vi "User Settings.vi"() -> ()   [LabVIEW 2025]
doc: "Access Level Admin only.\nFeature supported:\n1.Add User\n2.Change Password\n3.Remove User"
uses:
  <vilib>/addons/database/Connection.llb/Conn ObjectReference.ctl
  <vilib>/Utility/miscctls.llb/LVRectTypeDef.ctl
  <vilib>/Utility/error.llb/Trim Whitespace One-Sided.vi
  <vilib>/addons/database/NI_Database_API.lvlib
panel:
  in  "error in":errorcluster
  in  "User Configuration":string(tree)
  in  "Exit":bool
  in  "User Mangement":enum32{"Add", "Edit", "Delete"}(radio)
  in  "User_Tab":enum32{"Add", "Edit", "Delete"}(tab)
  in  "Add User":bool
  in  "Work Group":string(combo)="Operator"
  in  "Confirm Password":string
  in  "New Password":string
  in  "New User":string
  out "UserName Edit":string caption="UserName"
  in  "ChangeCONFIRMPassword":string caption="Confirm Password *"
  in  "ChangeNEWPassword":string caption="New Password *"
  in  "ChangeOldPassword":string caption="Current Password *"
  in  "Update User":bool
  in  "Remove User":bool
  out "UserName Delete":string caption="UserName"
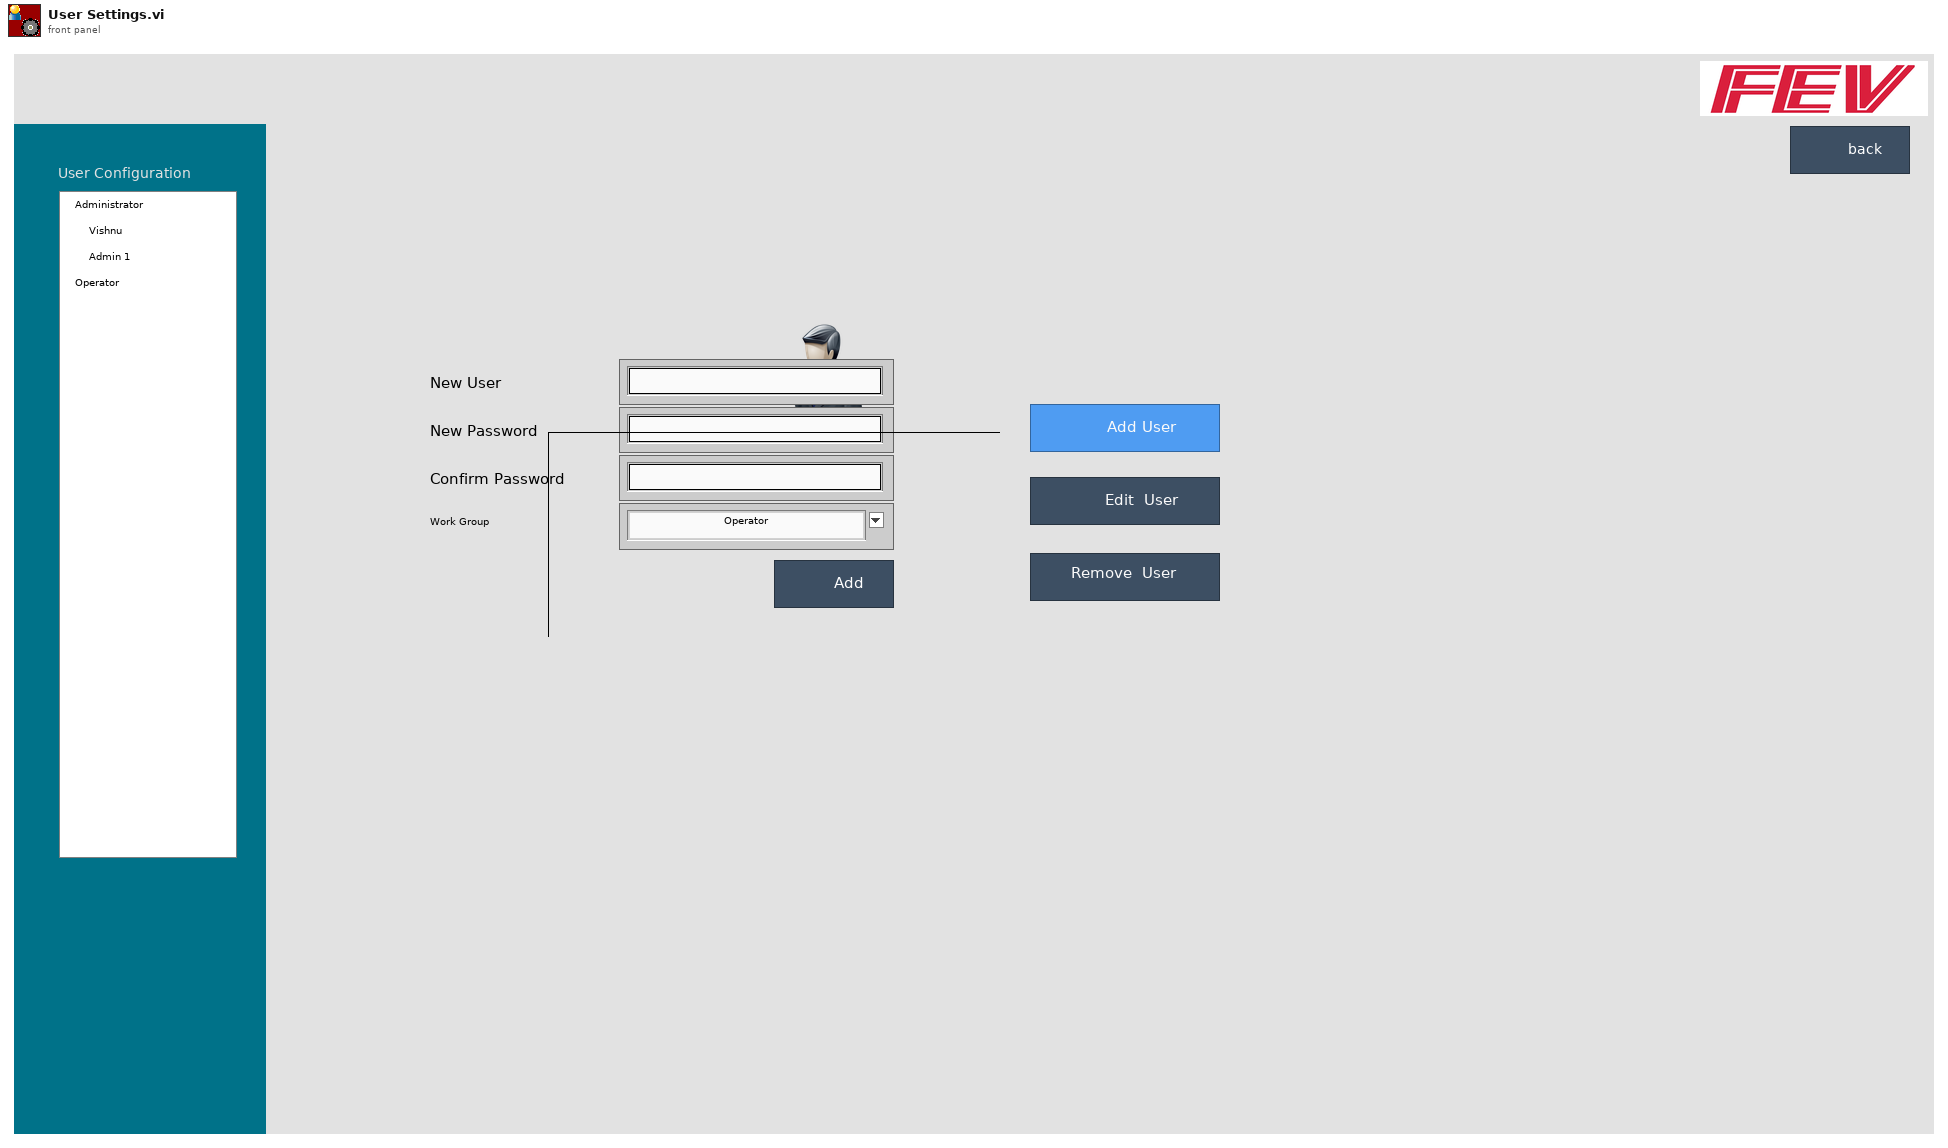
[diagram p1: front panel]
types:
  T1 = typedef "LVRectTypeDef.ctl" = cluster{"Left":i16, "Top":i16, "Right":i16, "Bottom":i16}
  T2 = typedef "NI_Database_API.lvlib/Conn ObjectReference.ctl" = refnum<k1>
  T3 = cluster{"UserDetails":string[][], "AcitveDBCon":T2}
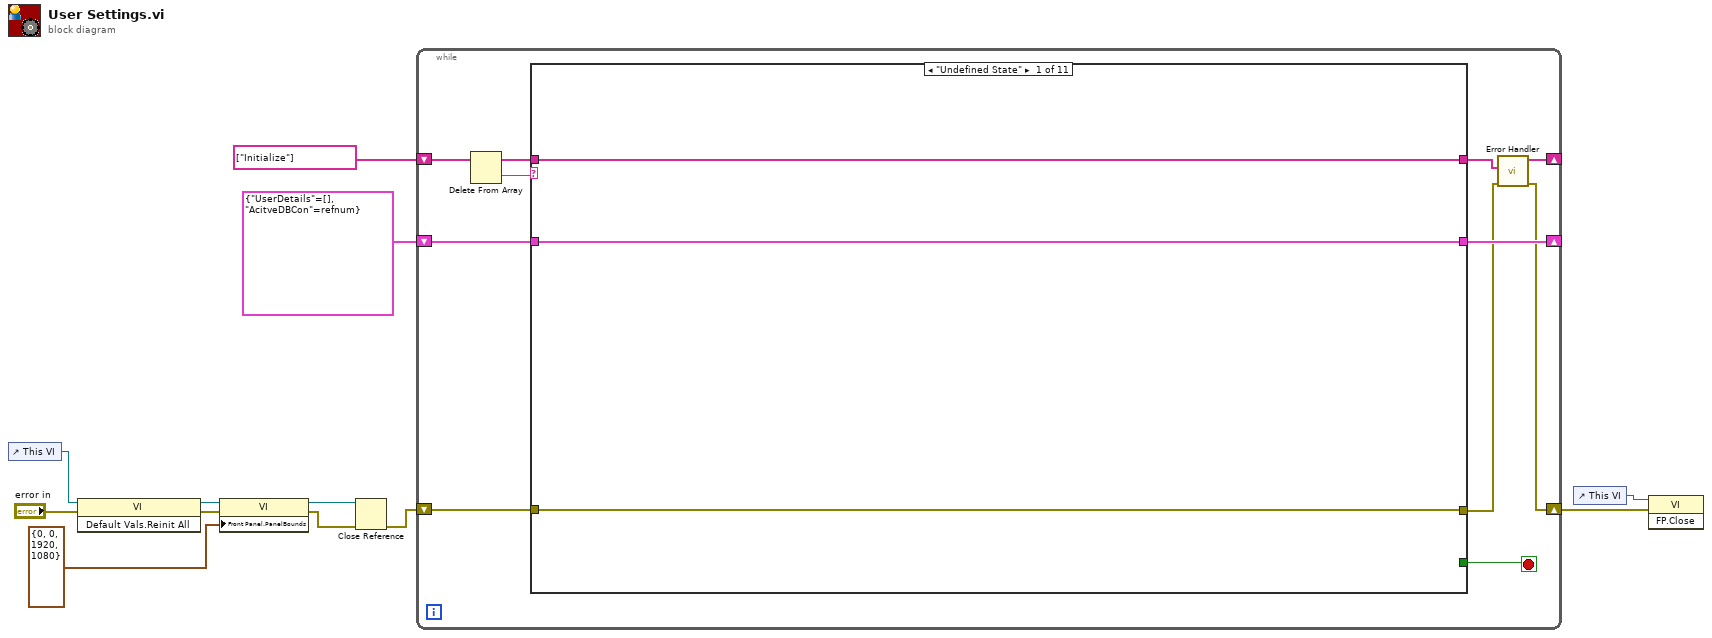
[diagram p0: block diagram]
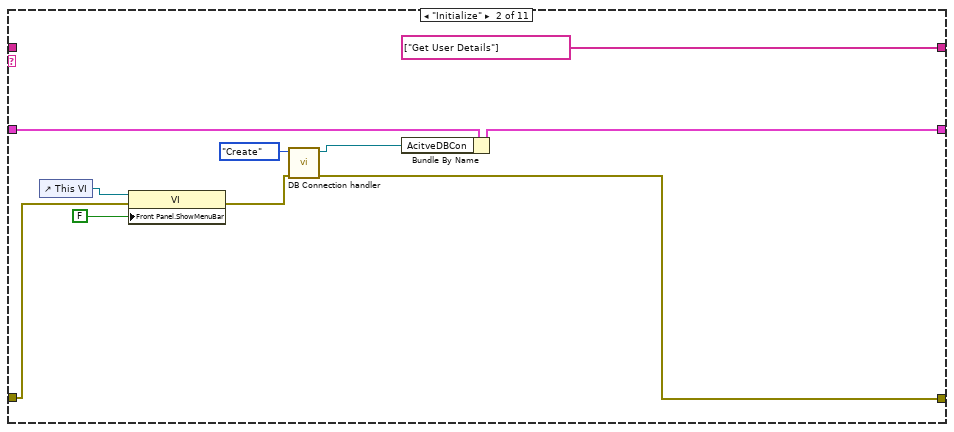
[diagram p2: hidden frame]
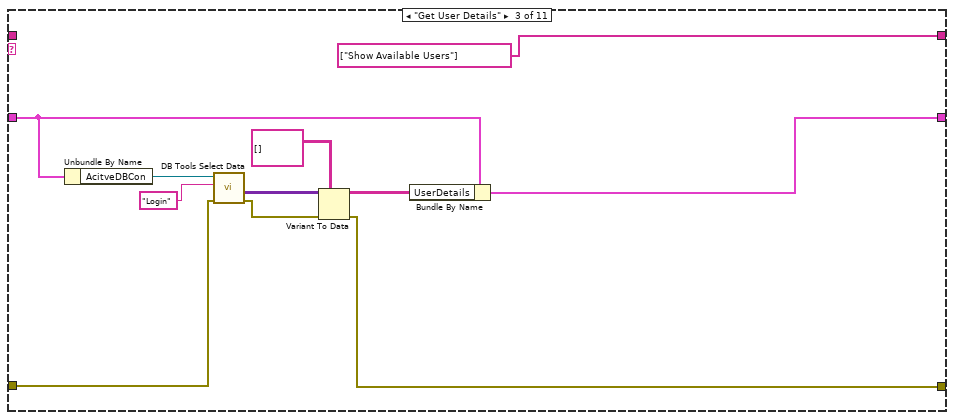
[diagram p3: hidden frame]
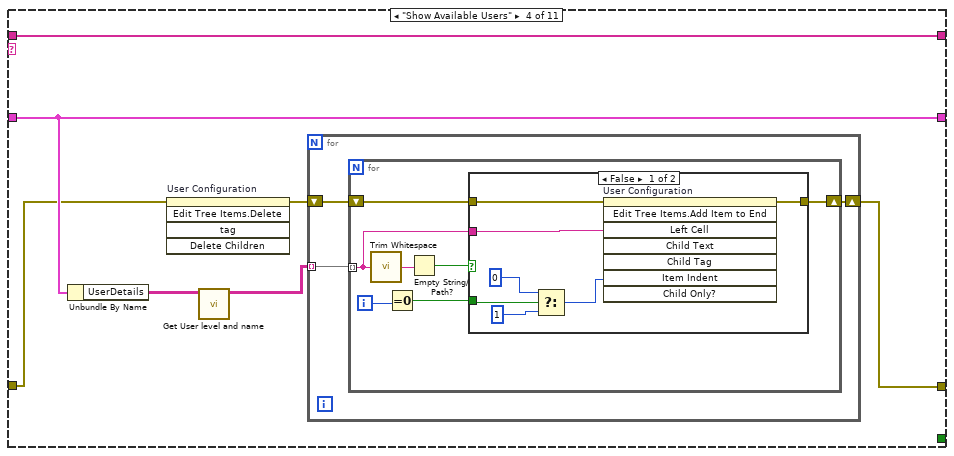
[diagram p4: hidden frame]
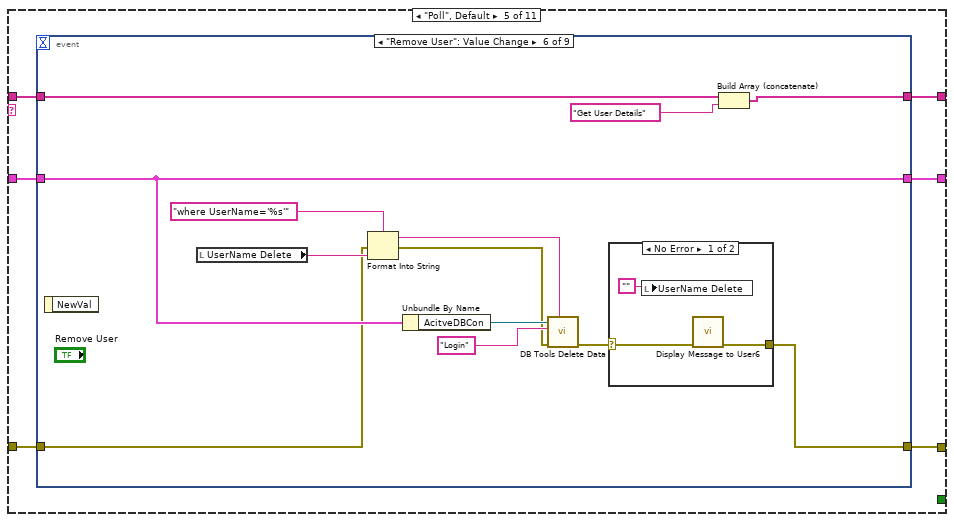
[diagram p6: hidden frame]
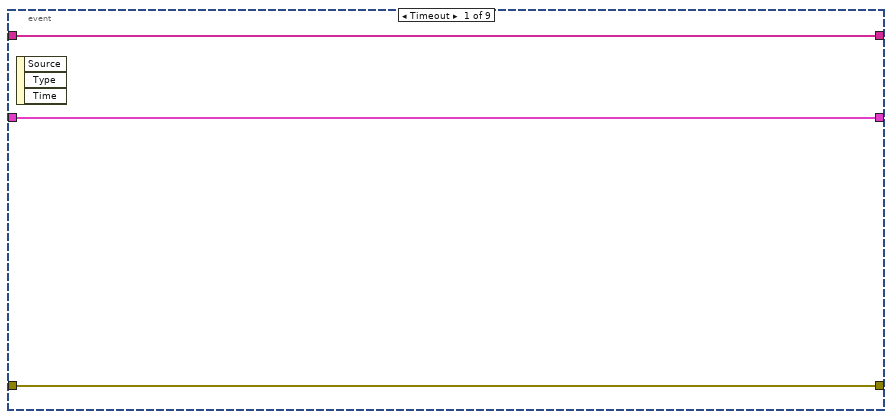
[diagram p7: hidden frame]
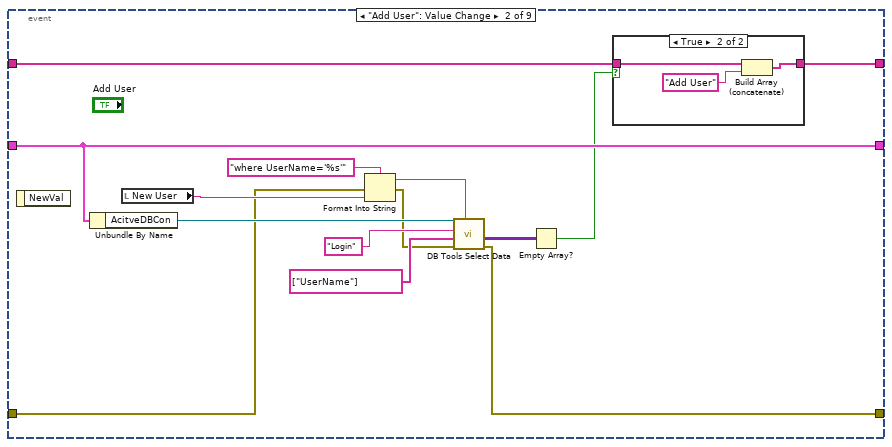
[diagram p8: hidden frame]
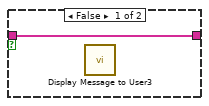
[diagram p9: hidden frame]
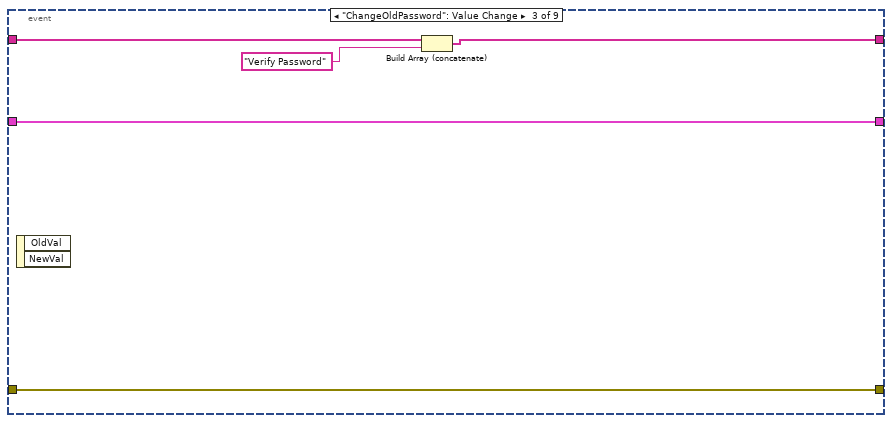
[diagram p10: hidden frame]
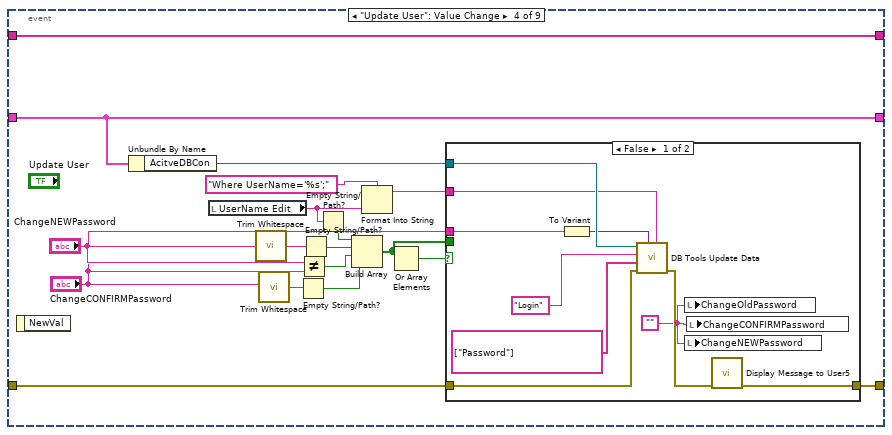
[diagram p11: hidden frame]
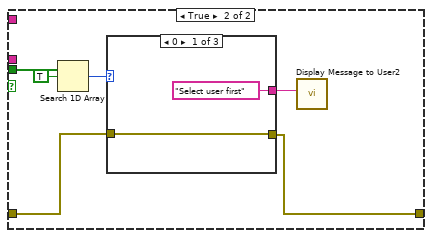
[diagram p12: hidden frame]
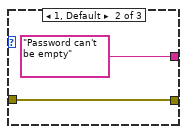
[diagram p13: hidden frame]
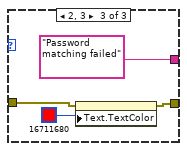
[diagram p14: hidden frame]
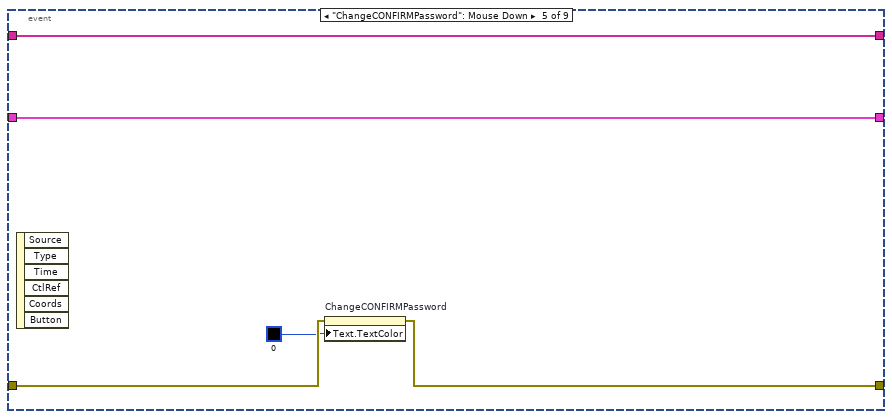
[diagram p15: hidden frame]
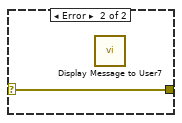
[diagram p16: hidden frame]
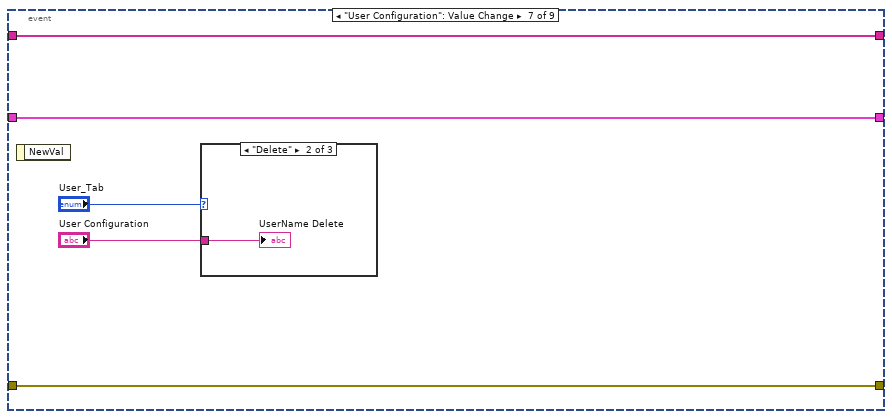
[diagram p17: hidden frame]
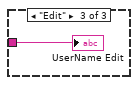
[diagram p19: hidden frame]
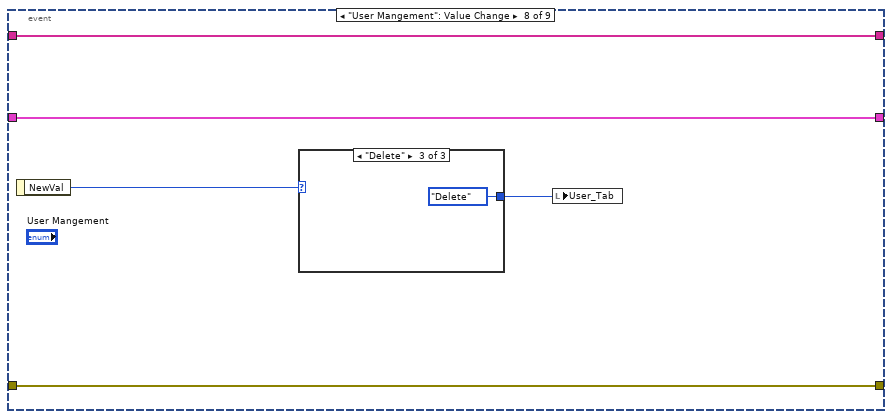
[diagram p20: hidden frame]
diagram:
  n1 = control-ref of="This VI"() -> (w6:refnum<vi>)
  n2 = invoke class="VI" method="Default Vals.Reinit All"(reference=w6, error in="error in") -> (reference out=w5:refnum<vi>, error out=w2:errorcluster)  [unwired: 1 in, 1 out]
  n3 = property class="VI"(reference=w5, error in=w2, "Front Panel.PanelBounds"=T1 {"Left"=0, "Top"=0, "Right"=1920, "Bottom"=1080} ("Front Panel Window:Window Bounds")) -> (reference out=w4:refnum<vi>, error out=w1:errorcluster)
  n4 = Close Reference(reference=w4, error in (no error)=w1) -> (error out=w11:errorcluster)
  n5 = while {
    shift-right: [w17] -> _
    shift-left: string[] ["Initialize"] -> [w22]
    shift-right: [w20] -> _
    shift-left: T3 {"UserDetails"=[], "AcitveDBCon"=refnum} -> [w19]
    shift-right: [w15] -> w7
    shift-left: w11 -> [w18]
    stop <- w14 stop-if-true
    n6 = Delete From Array(array=w22) -> (deleted portion=w23:string, array with subset deleted=w21:string[])  [unwired: 2 in]
    n7 = case shown="\"Undefined State\"" w23 {
      tunnel: [w26 string[] ["Get User Details"] string[] ["Show Available Users"] w54 w76 w192 w205 w223 w225 w240 w244] -> w13
      tunnel: w21 -> [w26 _ _ w54 w75 w200 w205 w223 w233 w240 w244]
      tunnel: [w25 w33 w46 w52 w78 w199 w217 w222 w232 w239 w243] -> w20
      tunnel: w19 -> [w25 w35 w45 w52 w77 w199 w217 w222 w232 w239 w243]
      tunnel: w18 -> [w24 w28 w38 w50 w73 w197 w213 w221 w227 w236 w241]
      tunnel: [w24 w31 w37 w53 w74 w189 w207 w221 w226 w234 w241] -> w16
      tunnel: [_ _ _ _ _ _ _ _ _ TRUE TRUE] -> w14
      frame "Undefined State" {
      }
      frame "Initialize" {
        n8 = control-ref of="This VI"() -> (w30:refnum<vi>)
        n9 = property class="VI"(reference=w30, error in=w28, "Front Panel.ShowMenuBar"=FALSE ("Front Panel Window:Show Menu Bar")) -> (error out=w27:errorcluster)  [unwired: 1 out]
        n10 = call "DB Connection handler.vi"("error in (no error)"=w27, "DB Action"=enum16{"Create", "Close", "Get"}."Create") -> ("error out"=w31:errorcluster, "connection reference"=w32:T2)  [unwired: 8 in]
        n11 = Bundle By Name(cluster=w35, "AcitveDBCon"=w32) -> (w33:T3)
      }
      frame "Get User Details" {
        n12 = Unbundle By Name(w45) -> ("AcitveDBCon"=w44:T2)
        n13 = call <vilib>:"DB Tools Select Data.vi"("error in (no error)"=w38, "table"="Login", "connection reference"=w44) -> ("error out"=w39:errorcluster, "data"=w41:variant[][])  [unwired: 3 in, 1 out]
        n14 = Variant To Data(error in=w39, type=string[][] [], Variant=w41) -> (data=w40:string[][], error out=w37:errorcluster)
        n15 = Bundle By Name(cluster=w45, "UserDetails"=w40) -> (w46:T3)
      }
      frame "Show Available Users" {
        n16 = Unbundle By Name(w52) -> ("UserDetails"=w49:string[][])
        n17 = invoke on="User Configuration" class="Tree (strict)" method="Edit Tree Items.Delete"(error in=w50) -> (error out=w51:errorcluster)  [unwired: 4 in, 4 out]
        n18 = call "Get User level and name.vi"("UserDetails"=w49) -> ("UserL&N"=w48:string[][])  [unwired: 10 in]
        n19 = for {
          tunnel: w48 -> [w55] mode=indexing
          shift-right: [w57] -> w53
          shift-left: w51 -> [w56]
          n20 = for {
            shift-right: [w64] -> w57
            shift-left: w56 -> [w63]
            tunnel: w55 -> [w60] mode=indexing
            i -> [w62]
            n21 = call <vilib>:"Trim Whitespace.vi"("string"=w60) -> ("trimmed string"=w59:string)  [unwired: 1 in]
            n22 = Equal To 0?(x=w62) -> (x = 0?=w61:bool)
            n23 = Empty String/Path?(string/path=w59) -> (empty?=w58:bool)
            n24 = case shown="False" w58 {
              tunnel: [w71 w72] -> w64
              tunnel: w63 -> [w70 w72]
              tunnel: w61 -> [w69 _]
              tunnel: w60 -> [w65 _]
              frame False {
                n25 = Select(t=0, s=w69, f=1) -> (s? t:f=w66:i32)
                n26 = invoke on="User Configuration" class="Tree (strict)" method="Edit Tree Items.Add Item to End"(error in=w70, "Left Cell"=w65, "Item Indent"=w66) -> (error out=w71:errorcluster)  [unwired: 5 in, 7 out]
              }
              frame True {
              }
            }
          }
        }
      }
      frame "Poll", Default {
        n27 = event shown="[5] \"Remove User\": Value Change" {
          selector: _ -> [_ _ _ _ _ _ _ _ _]
          dyn-events: _ -> [_ _ _ _ _ _ _ _ _]
          timeout: _ -> [_ _ _ _ _ _ _ _ _]
          tunnel: [w81 w93 w104 w118 w150 w163 w172 w178 w187] -> w78
          tunnel: w77 -> [w81 w93 w104 w118 w150 w163 w172 w178 w187]
          tunnel: [w80 w95 w103 w122 w151 w155 w173 w179 w185] -> w76
          tunnel: w75 -> [w80 w94 w100 w122 w151 w164 w173 w179 w188]
          tunnel: [w79 w84 w101 w115 w148 w152 w171 w180 w186] -> w74
          tunnel: w73 -> [w79 w86 w101 w116 w149 w157 w171 w180 w186]
          event Timeout {
            n28 = event-data() -> ()  [unwired: 1 in, 3 out]
          }
          event "Add User": Value Change {
            n29 = event-data() -> ()  [unwired: 1 in, 1 out]
            n30 = Unbundle By Name(w93) -> ("AcitveDBCon"=w92:T2)
            n31 = local read "New User"() -> (w88:string)
            n32 = Format Into String(format string="where UserName='%s'", error in=w86, w88) -> (resulting string=w87:string, error out=w85:errorcluster)  [unwired: 1 in]
            n33 = call <vilib>:"DB Tools Select Data.vi"("condition"=w87, "error in (no error)"=w85, "columns"=string[] ["UserName"], "table"="Login", "connection reference"=w92) -> ("error out"=w84:errorcluster, "data"=w83:variant[][])  [unwired: 1 in, 1 out]
            n34 = Empty Array?(array=w83) -> (empty?=w82:bool)
            n35 = case shown="True" w82 {
              tunnel: [w96 w99] -> w95
              tunnel: w94 -> [w96 w97]
              frame False {
                n36 = call "Display Message to User3"() -> ()  [unwired: 10 in, 2 out]
              }
              frame True {
                n37 = Build Array (concatenate)(w97, "Add User") -> (w99:string[])
              }
            }
          }
          event "ChangeOldPassword": Value Change {
            n38 = event-data() -> ()  [unwired: 1 in, 2 out]
            n39 = Build Array (concatenate)(w100, "Verify Password") -> (w103:string[])
          }
          event "Update User": Value Change {
            n40 = event-data() -> ()  [unwired: 1 in, 1 out]
            n41 = Unbundle By Name(w118) -> ("AcitveDBCon"=w117:T2)
            n42 = local read "UserName Edit"() -> (w105:string)
            n43 = call <vilib>:"Trim Whitespace.vi"("string"="ChangeNEWPassword") -> ("trimmed string"=w121:string)  [unwired: 1 in]
            n44 = call <vilib>:"Trim Whitespace.vi"("string"="ChangeCONFIRMPassword") -> ("trimmed string"=w120:string)  [unwired: 1 in]
            n45 = Empty String/Path?(string/path=w120) -> (empty?=w109:bool)
            n46 = Not Equal?(x="ChangeNEWPassword", y="ChangeCONFIRMPassword") -> (x != y?=w110:bool)
            n47 = Empty String/Path?(string/path=w121) -> (empty?=w111:bool)
            n48 = Empty String/Path?(string/path=w105) -> (empty?=w106:bool)
            n49 = Build Array(w106, w111, w110, w109) -> (w107:bool[])
            n50 = Format Into String(format string="Where UserName='%s';", w105) -> (resulting string=w113:string)  [unwired: 2 in, 1 out]
            n51 = Or Array Elements(Boolean array=w107) -> (logical OR=w108:bool)
            n52 = case shown="False" w108 {
              tunnel: w117 -> [w132 _]
              tunnel: w116 -> [w129 w134]
              tunnel: [w124 w133] -> w115
              tunnel: "ChangeCONFIRMPassword" -> [w128 _]
              tunnel: w113 -> [w127 _]
              tunnel: w107 -> [_ w138]
              frame False {
                w123 = ""
                n53 = To Variant(anything=w128) -> (Variant=w126:variant)
                n54 = call <vilib>:"DB Tools Update Data.vi"("condition"=w127, "data"=w126, "error in (no error)"=w129, "columns"=string[] ["Password"], "table"="Login", "connection reference"=w132) -> ("error out"=w125:errorcluster)  [unwired: 4 in, 1 out]
                n55 = local write "ChangeOldPassword"(w123) -> ()
                n56 = local write "ChangeNEWPassword"(w123) -> ()
                n57 = local write "ChangeCONFIRMPassword"(w123) -> ()
                n58 = call "Display Message to User5"("error in (no error)"=w125) -> ("error out"=w124:errorcluster)  [unwired: 9 in, 1 out]
              }
              frame True {
                n59 = Search 1D Array(1D array=w138, element=TRUE) -> (index of element=w136:i32)  [unwired: 1 in]
                n60 = case shown="0" w136 {
                  tunnel: ["Select user first" "Password can't be empty" "Password matching failed"] -> w135
                  tunnel: w134 -> [w140 w141 w144]
                  tunnel: [w140 w141 w143] -> w133
                  frame 0 {
                  }
                  frame 1, Default {
                  }
                  frame 2, 3 {
                    n61 = property on="ChangeCONFIRMPassword" class="Str"(error in=w144, "Text.TextColor"=u32 16711680) -> (error out=w143:errorcluster)  [unwired: 1 in, 1 out]
                  }
                }
                n62 = call "Display Message to User2"("Message"=w135) -> ()  [unwired: 9 in, 2 out]
              }
            }
          }
          event "ChangeCONFIRMPassword": Mouse Down {
            n63 = event-data() -> ()  [unwired: 1 in, 6 out]
            n64 = property on="ChangeCONFIRMPassword" class="Str"(error in=w149, "Text.TextColor"=u32 0) -> (error out=w148:errorcluster)  [unwired: 1 in, 1 out]
          }
          event "Remove User": Value Change {
            n65 = event-data() -> ()  [unwired: 1 in, 1 out]
            n66 = local read "UserName Delete"() -> (w159:string)
            n67 = Format Into String(format string="where UserName='%s'" ("condition"), error in=w157, w159) -> (resulting string=w158:string, error out=w156:errorcluster)  [unwired: 1 in]
            n68 = Unbundle By Name(w163) -> ("AcitveDBCon"=w162:T2)
            n69 = call <vilib>:"DB Tools Delete Data.vi"("condition"=w158, "error in (no error)"=w156, "table"="Login", "connection reference"=w162) -> ("error out"=w153:errorcluster)  [unwired: 6 in, 1 out]
            n70 = case shown="No Error" w153 {
              selector: w153 -> [w167 w168]
              tunnel: [w166 w168] -> w152
              frame No Error {
                n71 = local write "UserName Delete"("") -> ()
                n72 = call "Display Message to User6"("error in (no error)"=w167) -> ("error out"=w166:errorcluster)  [unwired: 9 in, 1 out]
              }
              frame Error {
                n73 = call "Display Message to User7"() -> ()  [unwired: 10 in, 2 out]
              }
            }
            n74 = Build Array (concatenate)(w164, "Get User Details") -> (w155:string[])
          }
          event "User Configuration": Value Change {
            n75 = event-data() -> ()  [unwired: 1 in, 1 out]
            n76 = case shown="\"Delete\"" "User_Tab" {
              tunnel: "User Configuration" -> [_ w174 w175]
              frame "Add", Default {
              }
              frame "Delete" {
                "UserName Delete" <- w174
              }
              frame "Edit" {
                "UserName Edit" <- w175
              }
            }
          }
          event "User Mangement": Value Change {
            n77 = event-data() -> ("NewVal"=w177:enum32{"Add", "Edit", "Delete"})  [unwired: 1 in]
            n78 = case shown="\"Delete\"" w177 {
              tunnel: [enum32{"Add", "Edit", "Delete"}."Add" ("User_Tab") enum32{"Add", "Edit", "Delete"}."Edit" ("User_Tab") enum32{"Add", "Edit", "Delete"}."Delete" ("User_Tab")] -> w176
              frame "Add", Default {
              }
              frame "Edit" {
              }
              frame "Delete" {
              }
            }
            n79 = local write "User_Tab"(w176) -> ()
          }
          event "Exit": Value Change {
            n80 = event-data() -> ()  [unwired: 1 in, 6 out]
            n81 = Build Array (concatenate)(w188, "Exit") -> (w185:string[])
          }
        }
      }
      frame "Add User" {
        n82 = Unbundle By Name(w199) -> ("AcitveDBCon"=w198:T2)
        n83 = call "Add User.vi"("New Password"="New Password", "New User"="New User", "error in (no error)"=w197, "Confirm Password"="Confirm Password", "Work Group"="Work Group", "Refnum in"=w198) -> ("error out"=w190:errorcluster)  [unwired: 5 in]
        n84 = Build Array (concatenate)(w200, "Get User Details") -> (w192:string[])
        n85 = flat-sequence {
          tunnel: w190 -> [w201]
          tunnel: [w201] -> w189
          frame #0 {
            w202 = ""
            n86 = local write "New User"(w202) -> ()
            n87 = local write "New Password"(w202) -> ()
            n88 = local write "Confirm Password"(w202) -> ()
          }
        }
      }
      frame "Verify Password" {
        n89 = local read "UserName Edit"() -> (w211:string)
        n90 = Unbundle By Name(w217) -> ("AcitveDBCon"=w216:T2)
        n91 = Format Into String(format string="where UserName='%s' and Password='%s' ", error in=w213, w211, "ChangeOldPassword") -> (resulting string=w206:string, error out=w212:errorcluster)  [unwired: 1 in]
        n92 = call <vilib>:"DB Tools Select Data.vi"("condition"=w206, "error in (no error)"=w212, "table"="Login", "connection reference"=w216) -> ("error out"=w208:errorcluster, "data"=w210:variant[][], "connection reference out"=w204:T2)  [unwired: 2 in]
        n93 = Empty Array?(array=w210) -> (empty?=w209:bool)
        n94 = case shown="False" w209 {
          tunnel: w208 -> [w218 w220]
          tunnel: [w218 w219] -> w207
          tunnel: w204 -> [_ _]
          frame False {
          }
          frame True {
            n95 = call "Display Message to User"("error in (no error)"=w220) -> ("error out"=w219:errorcluster)  [unwired: 9 in, 1 out]
          }
        }
      }
      frame "Update Details" {
      }
      frame "Launch Home Screen" {
        n96 = call <vilib>:"Application Directory.vi"() -> ("Application Directory"=w230:path)
        n97 = Build Path(base path=w230, name or relative path="Test Module\\Home Screen.vi") -> (appended path=w228:path)
        n98 = call "Run VI Dynamically2.vi"("error in (no error)"=w227, "Show FP?"=TRUE ("Show FP"), "Vi Path"=w228) -> ("error out"=w226:errorcluster)  [unwired: 7 in, 1 out]
        n99 = Build Array (concatenate)(w233, "Exit") -> (w225:string[])
      }
      frame "Exit on Error" {
        n100 = Unbundle By Name(w236) -> ("source"=w237:string)
        n101 = call <vilib>:"Clear Errors.vi"("error in (no error)"=w236) -> ("error out"=w235:errorcluster)  [unwired: 5 in, 1 out]
        n102 = call "Display Message to User4"("error in (no error)"=w235, "Message"=w237) -> ("error out"=w234:errorcluster)  [unwired: 8 in, 1 out]
      }
      frame "Exit" {
      }
    }
    n103 = call "Error Handler.vi"("error in (no error)"=w16, "States In"=w13) -> ("error out"=w15:errorcluster, "States Out"=w17:string[])  [unwired: 8 in]
  }
  n104 = control-ref of="This VI"() -> (w8:refnum<vi>)
  n105 = invoke class="VI" method="FP.Close"(reference=w8, error in=w7) -> ()  [unwired: 1 in, 3 out]
